vi "VALEW_Sensors_Pressure.vi"(0 "GEA2 Reference In":refnum<k24>, 1 "Lim_L_Pressure ADC Count":dbl[](array[numeric])=[0.0, 755.0, 1560.0, 2350.0, 3165.0, 3970.0], 3 "Lim_U_Pressure ADC Count":dbl[](array[numeric])=[50.0, 855.0, 1660.0, 2450.0, 3265.0, 4070.0], 5 "GEA Inputs":T1={"Source"=228, "Destination"=35} {"Destination" format="%.0x"; "Source" format="%.0x"}, 7 "DAQmx Physical Channel":tag="9269_1/ao0", 9 "Array of Voltages":dbl[](array[numeric])=[0.0, 1.0, 2.0, 3.0, 4.0, 5.0], 10 "Standalone?":bool, 11 "Error In":errorcluster, 12 "Lim_L_Pressure (inches of water)":dbl[](array[numeric])=[0.0, 2.2, 7.14, 12.2, 17.25, 19.8], 14 "Lim_U_Pressure (inches of water)":dbl[](array[numeric])=[0.0, 2.6, 7.44, 12.6, 17.55, 20.2]) -> (2 "Pressure ADC Count":dbl[](array[numeric])=[1.0, 805.0, 1609.0, 2413.0, 3216.0, 4021.0], 4 "GEA2 Reference Out":refnum<k24>, 6 "Pass/Fail?":bool, 8 "Report Text":string, 13 "Pressure (inches of water)":dbl[](array[numeric])=[0.0, 2.413, 7.338, 12.262, 17.187, 20.066], 15 "Error Out":errorcluster={"status"=TRUE, "code"=-5002, "source"="Verify Results - Upper and Lower Limit.vi<ERR>\nUpper Limit, Lower Limit, and Results Arrays must all be equal size and not be zero.\n\n\n<b>Complete call chain:</b>\r\n     Verify Results - Upper and Lower Limit.vi\r\n     VALEW_Sensors_Pressure.vi\r\n     VALEW_Sensors_Pressure.vi.ProxyCaller"})   [LabVIEW 2016, in "Centauro.lvlib"]
uses:
  Projects/Centauro.lvlib
  Q:/Common/DLLs/GEA3/GeaCommunication.dll
  Common/DLLs/GEA3/GeaCommunication.dll
  Common/LabVIEW GEA2 Toolkit/LabVIEW_GEA2_Toolkit.lvlibp/type defs/Source_Destination.ctl
  Common/LabVIEW GEA2 Toolkit/LabVIEW_GEA2_Toolkit.lvlibp/type defs/ERD Write Data In.ctl
  Common/LabVIEW GEA2 Toolkit/LabVIEW_GEA2_Toolkit.lvlibp/type defs/Data Type.ctl
  Common/LabVIEW GEA2 Toolkit/LabVIEW_GEA2_Toolkit.lvlibp/type defs/ERD Read Data In.ctl
  <vilib>/DAQmx/write.llb/DAQmx Write (Analog DBL 1Chan 1Samp).vi
  <vilib>/DAQmx/create/channels.llb/DAQmx Create Channel (AO-Voltage-Basic).vi
  <vilib>/DAQmx/miscellaneous.llb/DAQmx Fill In Error Info.vi
  Common/LabVIEW GEA2 Toolkit/LabVIEW_GEA2_Toolkit.lvlibp
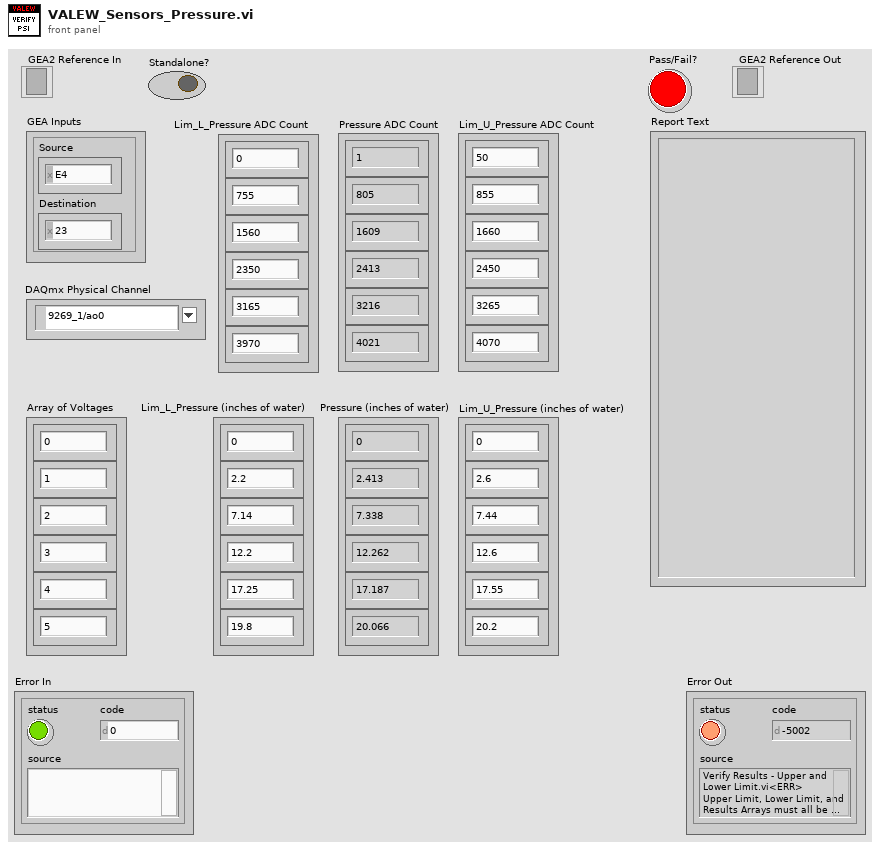
[diagram p1: front panel]
types:
  T1 = typedef "LabVIEW_GEA2_Toolkit.lvlibp/Source_Destination.ctl" = cluster{"Source":u8, "Destination":u8}
  T2 = typedef "LabVIEW_GEA2_Toolkit.lvlibp/ERD Write Data In.ctl" = cluster{"ERD Number":u16, "Data Type":T3, "Data":string}
  T3 = typedef "LabVIEW_GEA2_Toolkit.lvlibp/Data Type.ctl" = enum16{"string", "boolean", "uint8_t", "uint16_t", "uint32_t", "uint64_t", "int8_t", "int16_t", "int32_t", "int64_t"}
  T4 = typedef "LabVIEW_GEA2_Toolkit.lvlibp/ERD Read Data In.ctl" = cluster{"ERD Number":u16, "Data Type":T3}
  T5 = typedef "LabVIEW_GEA2_Toolkit.lvlibp/ERD Read Data Out.ctl" = cluster{"ERD Number":u16, "Data":string}
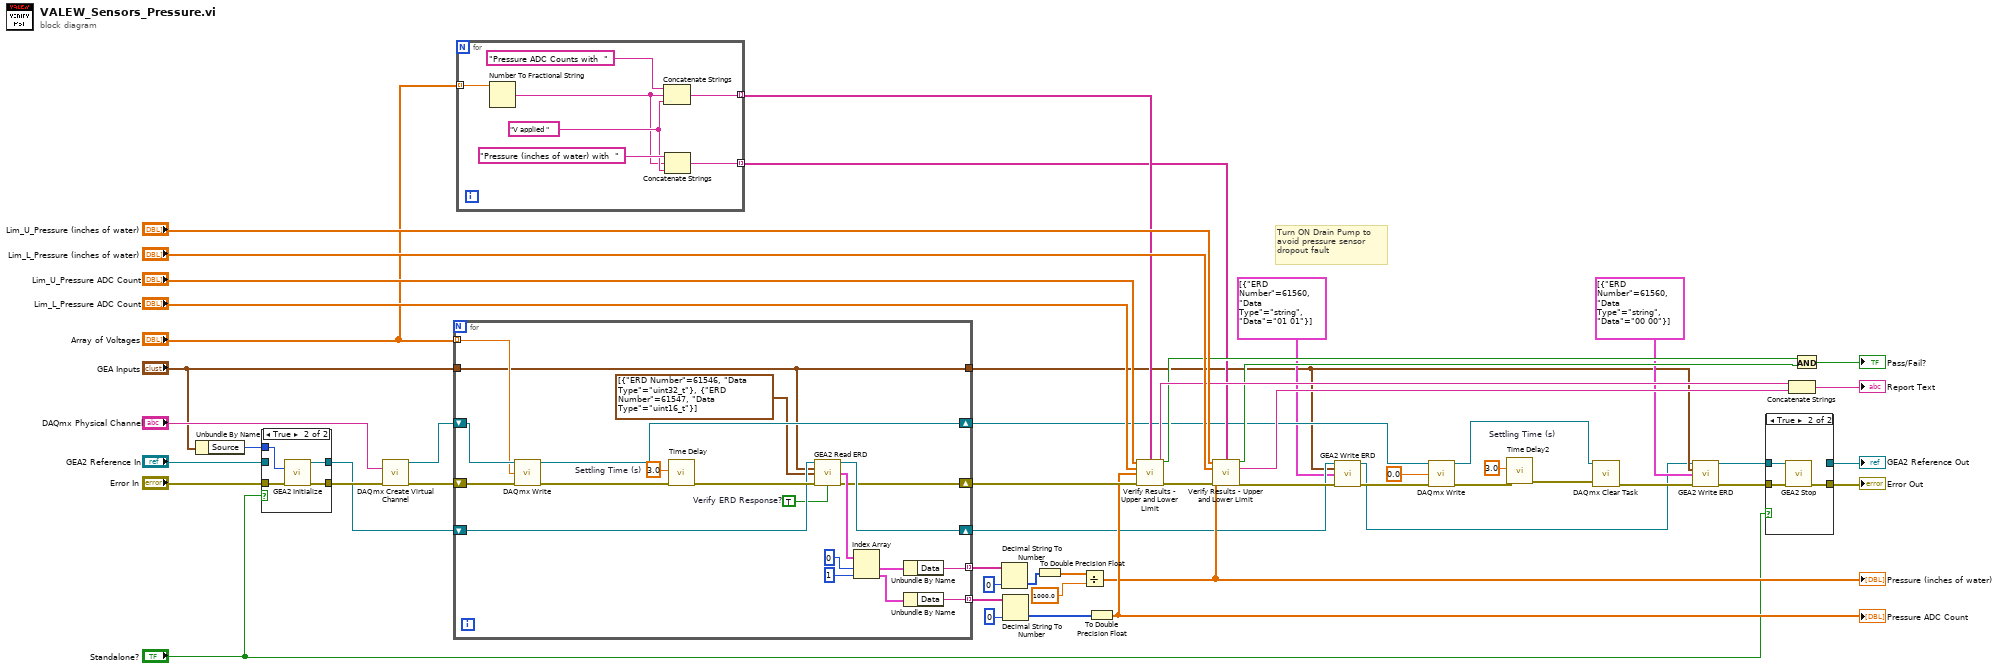
[diagram p0: block diagram]
diagram:
  w14 = 3.0  # Settling Time (s)
  # "Turn ON Drain Pump to \navoid pressure sensor \ndropout fault"
  n1 = Unbundle By Name("GEA Inputs") -> ("Source"=w45:u8)
  n2 = case shown="True" "Standalone?" {
    tunnel: "Error In" -> [w55 w59]
    tunnel: [w55 w58] -> w50
    tunnel: "GEA2 Reference In" -> [w54 _]
    tunnel: [w54 w57] -> w46
    tunnel: w45 -> [_ w56]
    frame False {
    }
    frame True {
      n3 = call "GEA2 Initialize.vi"("Source Address"=w56, "error in"=w59) -> ("GEA2 Reference Out"=w57:refnum<k24>, "error out"=w58:errorcluster)  [unwired: 11 in, 1 out]
    }
  }
  n4 = call-poly <vilib>:"DAQmx Create Virtual Channel.vi"("physical channels"="DAQmx Physical Channel", "error in"=w50) -> ("task out"=w48:refnum<k21>, "error out"=w49:errorcluster)  [unwired: 12 in]
  n5 = for {
    shift-right: [w62] -> w9
    shift-left: w46 -> [w73]
    shift-right: [w78] -> w16
    shift-left: w48 -> [w77]
    shift-right: [w61] -> w38
    shift-left: w49 -> [w79]
    tunnel: "GEA Inputs" -> [w60]
    tunnel: "Array of Voltages" -> [w72] mode=indexing
    tunnel: [w69] -> w43 mode=indexing
    tunnel: [w68] -> w40 mode=indexing
    tunnel: [w60] -> w4
    w67 = TRUE  # Verify ERD Response?
    w76 = 3.0  # Settling Time (s)
    n6 = call-poly <vilib>:"DAQmx Write.vi"("task/channels in"=w77, "data"=w72, "error in"=w79) -> ("task out"=w78:refnum<k21>, "error out"=w74:errorcluster)  [unwired: 10 in, 1 out]
    n7 = call "Time Delay"("error in (no error)"=w74, "Delay Time (s)"=w76) -> ("error out"=w75:errorcluster)  [unwired: 9 in]
    n8 = call "GEA2 Read ERD.vi"("GEA2 Reference In"=w73, "GEA Inputs"=w60, "Read ERD List"=T4[] [{"ERD Number"=61546, "Data Type"=enum."uint32_t"}, {"ERD Number"=61547, "Data Type"=enum."uint16_t"}], "Error In"=w75, "Verify ERD Response?"=w67) -> ("GEA2 Reference Out"=w62:refnum<k24>, "ERD Data Out"=w71:T5[], "Error Out"=w61:errorcluster)  [unwired: 7 in, 1 out]
    n9 = Index Array(array=w71, index #1=0 ("index"), index #2=1 ("index")) -> (element #1=w65:T5, element #2=w64:T5)
    n10 = Unbundle By Name(w65) -> ("Data"=w68:string)
    n11 = Unbundle By Name(w64) -> ("Data"=w69:string)
  }
  n12 = for {
    tunnel: "Array of Voltages" -> [w86] mode=indexing
    tunnel: [w81] -> w19 mode=indexing
    tunnel: [w80] -> w20 mode=indexing
    w83 = "V applied "
    n13 = Number To Fractional String(number=w86) -> (F-format string=w82:string)  [unwired: 3 in]
    n14 = Concatenate Strings("Pressure ADC Counts with  ", w82, w83) -> (w80:string)
    n15 = Concatenate Strings("Pressure (inches of water) with  ", w82, w83) -> (w81:string)
  }
  n16 = Decimal String To Number(string=w40, default (0L)=u32 0 ("default (0 I32)")) -> (number=w33:u32[])  [unwired: 1 in, 1 out]
  n17 = Decimal String To Number(string=w43, default (0L)=u16 0 ("default (0 I32)")) -> (number=w37:u16[])  [unwired: 1 in, 1 out]
  n18 = To Double Precision Float(number=w33) -> (double precision float=w34:dbl[])
  n19 = Divide(x=w34, y=1000.0) -> (x/y=w32:dbl[])
  "Pressure (inches of water)" <- w32
  n20 = To Double Precision Float(number=w37) -> (double precision float=w36:dbl[])
  "Pressure ADC Count" <- w36
  n21 = call "Verify Results - Upper and Lower Limit.vi"("Upper Limits"="Lim_U_Pressure ADC Count", "Array of Names"=w20, "Lower Limits"="Lim_L_Pressure ADC Count", "Results"=w36, "Error In"=w38) -> ("Pass/Fail?"=w22:bool, "Report Text"=w26:string, "Error Out"=w39:errorcluster)  [unwired: 7 in, 1 out]
  n22 = call "Verify Results - Upper and Lower Limit.vi"("Upper Limits"="Lim_U_Pressure (inches of water)", "Array of Names"=w19, "Lower Limits"="Lim_L_Pressure (inches of water)", "Results"=w32, "Error In"=w39) -> ("Pass/Fail?"=w23:bool, "Report Text"=w27:string, "Error Out"=w17:errorcluster)  [unwired: 7 in, 1 out]
  n23 = call "GEA2 Write ERD.vi"("GEA2 Reference In"=w9, "GEA Inputs"=w4, "Write ERD List"=T2[] [{"ERD Number"=61560, "Data Type"=enum."string", "Data"="01 01"}], "Error In"=w17) -> ("GEA2 Reference Out"=w3:refnum<k24>, "Error Out"=w10:errorcluster)  [unwired: 9 in, 1 out]
  n24 = call-poly <vilib>:"DAQmx Write.vi"("task/channels in"=w16, "data"=0.0, "error in"=w10) -> ("task out"=w11:refnum<k21>, "error out"=w13:errorcluster)  [unwired: 10 in, 1 out]
  n25 = call "Time Delay2"("error in (no error)"=w13, "Delay Time (s)"=w14) -> ("error out"=w12:errorcluster)  [unwired: 9 in]
  n26 = call <vilib>:"DAQmx Clear Task.vi"("task in"=w11, "error in"=w12) -> ("error out"=w6:errorcluster)  [unwired: 13 in]
  n27 = call "GEA2 Write ERD.vi"("GEA2 Reference In"=w3, "GEA Inputs"=w4, "Write ERD List"=T2[] [{"ERD Number"=61560, "Data Type"=enum."string", "Data"="00 00"}], "Error In"=w6) -> ("GEA2 Reference Out"=w2:refnum<k24>, "Error Out"=w5:errorcluster)  [unwired: 9 in, 1 out]
  n28 = case shown="True" "Standalone?" {
    tunnel: [w88 w91] -> w47
    tunnel: w5 -> [w88 w90]
    tunnel: w2 -> [w87 w89]
    tunnel: [w87 _] -> w1
    frame False {
    }
    frame True {
      n29 = call "GEA2 Stop.vi"("GEA2 Reference In"=w89, "Error In"=w90) -> ("Error Out"=w91:errorcluster)  [unwired: 13 in]
    }
  }
  "Error Out" <- w47
  "GEA2 Reference Out" <- w1
  n30 = Concatenate Strings(w26, w27) -> (→"Report Text":string)
  n31 = And(x=w22, y=w23) -> (x .and. y?=→"Pass/Fail?":bool)
